vi "Mérésképernyő UI engedélyezés.vi"(8 "Error In":errorcluster, 10 "Felhasználói szint":string, 11 "UI Data":T1) -> (0 "Error Out":errorcluster, 3 "UI Data out":T1)   [LabVIEW 2014]
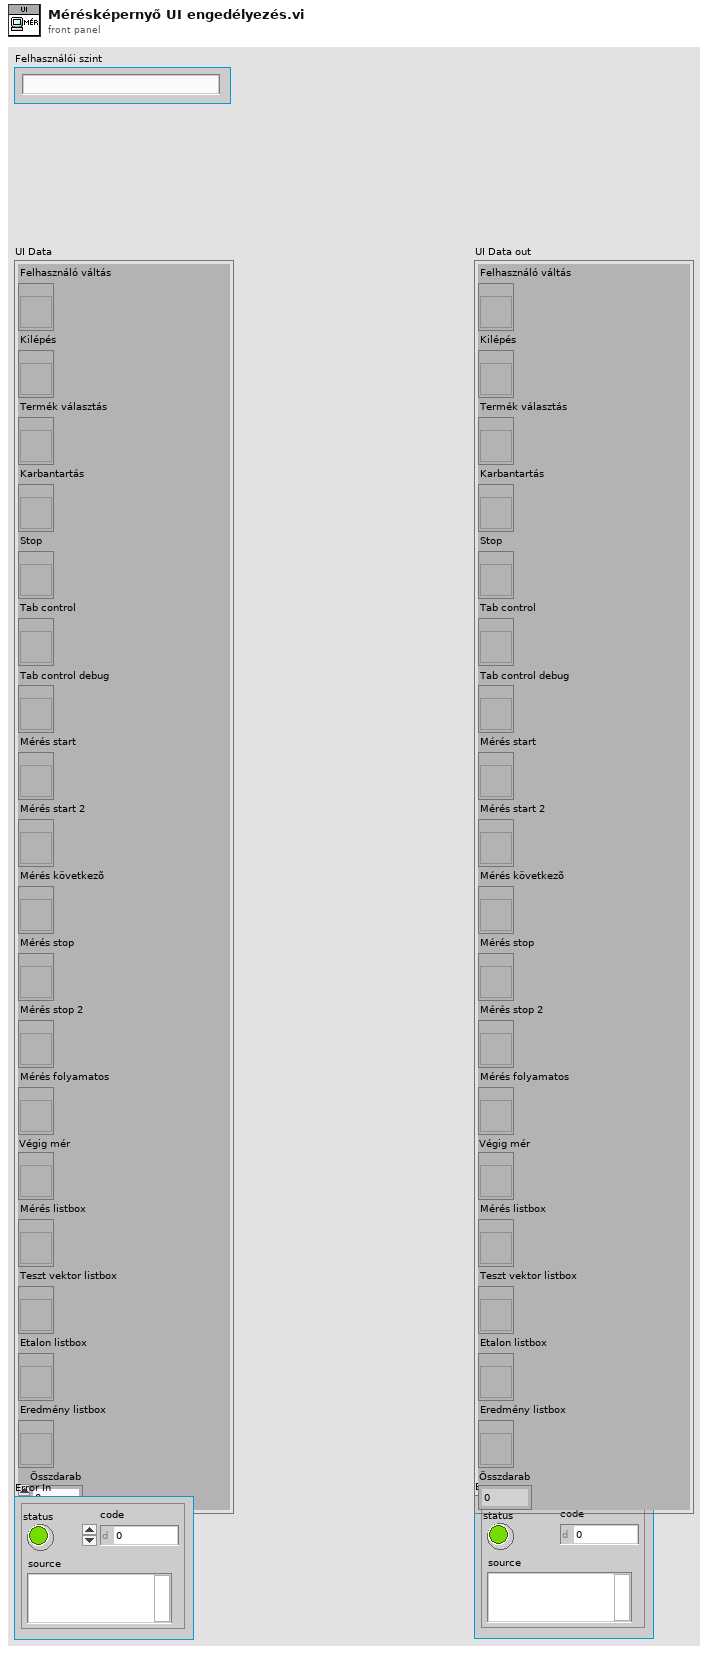
[diagram p1: front panel]
types:
  T1 = typedef "Fõképernyõ references.ctl" = cluster{"Felhasználó váltás":refnum<vi>, "Kilépés":refnum<vi>, "Termék választás":refnum<vi>, "Karbantartás":refnum<vi>, "Stop":refnum<vi>, "Tab control":refnum<vi>, "Tab control debug":refnum<vi>, "Mérés start":refnum<vi>, "Mérés start 2":refnum<vi>, "Mérés következõ":refnum<vi>, "Mérés stop":refnum<vi>, "Mérés stop 2":refnum<vi>, "Mérés folyamatos":refnum<vi>, "Végig mér":refnum<vi>, "Mérés listbox":refnum<vi>, "Teszt vektor listbox":refnum<vi>, "Etalon listbox":refnum<vi>, "Eredmény listbox":refnum<vi>, "Összdarab":i64}
  T2 = enum8{"Enabled", "Disabled", "Disabled and Grayed Out"}
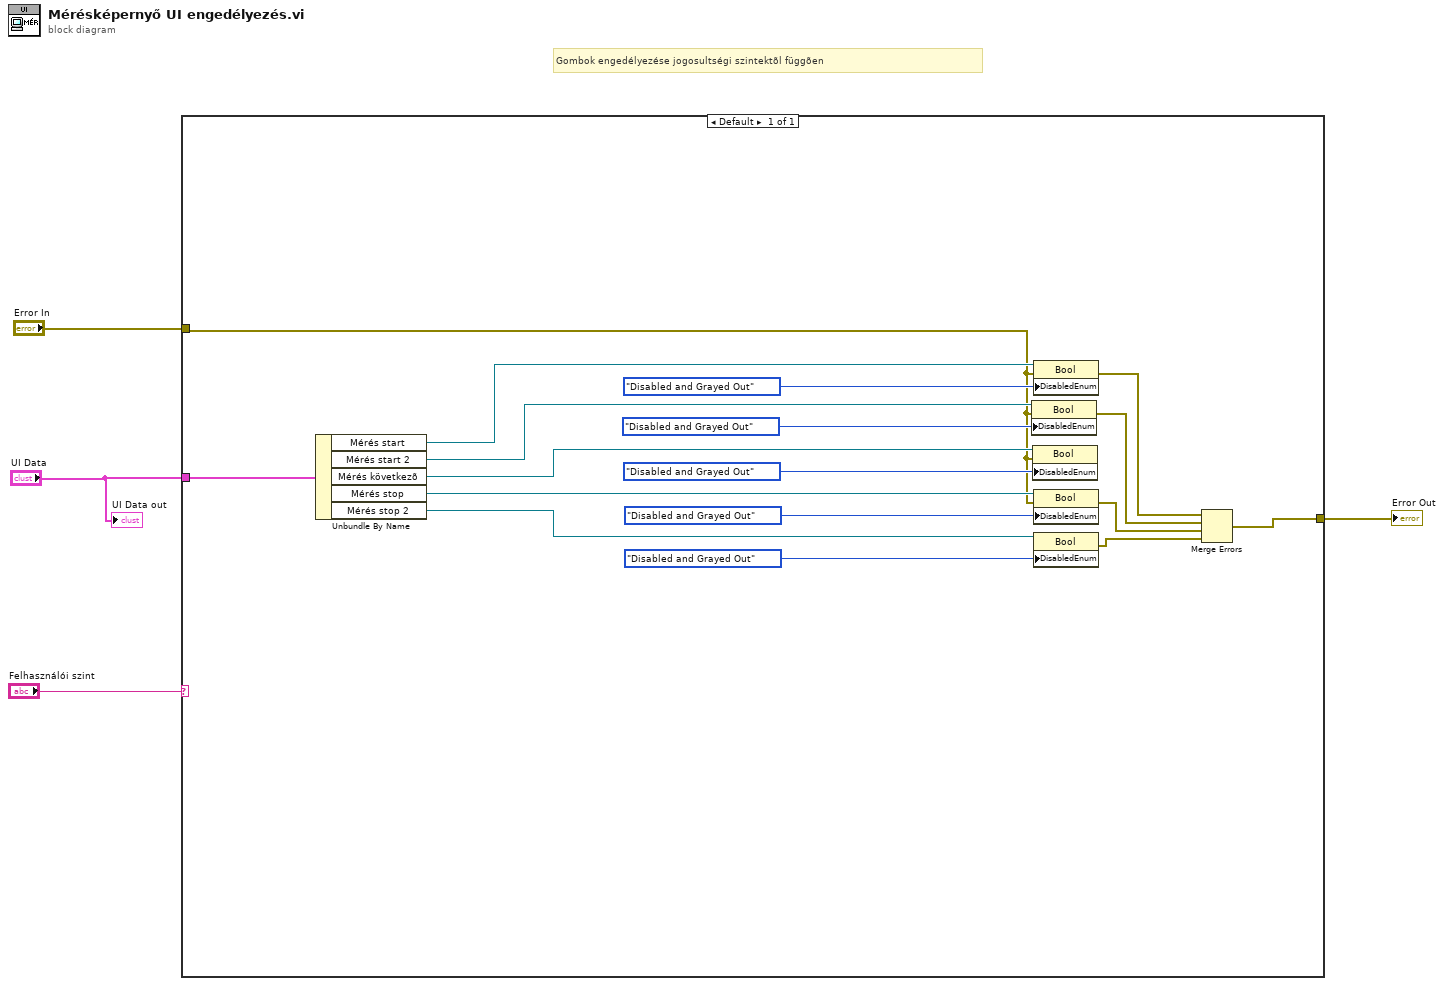
[diagram p0: block diagram]
diagram:
  # "Gombok engedélyezése jogosultségi szintektõl függõen"
  n1 = case shown="Default" "Felhasználói szint" {
    tunnel: [w10] -> w4
    tunnel: "UI Data" -> [w8]
    tunnel: "Error In" -> [w9]
    frame Default {
      n2 = Unbundle By Name(w8) -> ("Mérés start"=w19:refnum<vi>, "Mérés start 2"=w18:refnum<vi>, "Mérés következõ"=w17:refnum<vi>, "Mérés stop"=w15:refnum<vi>, "Mérés stop 2"=w6:refnum<vi>)
      n3 = property on="Property Node" class="Bool"(reference=w18, error in=w9, "DisabledEnum"=T2."Disabled and Grayed Out" ("Disabled")) -> (error out=w12:errorcluster)  [unwired: 1 out]
      n4 = property on="Property Node" class="Bool"(reference=w17, error in=w9, "DisabledEnum"=T2."Disabled and Grayed Out" ("Disabled")) -> ()  [unwired: 2 out]
      n5 = property on="Property Node" class="Bool"(reference=w19, error in=w9, "DisabledEnum"=T2."Disabled and Grayed Out" ("Disabled")) -> (error out=w13:errorcluster)  [unwired: 1 out]
      n6 = property on="Property Node" class="Bool"(reference=w15, error in=w9, "DisabledEnum"=T2."Disabled and Grayed Out" ("Disabled")) -> (error out=w11:errorcluster)  [unwired: 1 out]
      n7 = property on="Property Node" class="Bool"(reference=w6, "DisabledEnum"=T2."Disabled and Grayed Out" ("Disabled")) -> (error out=w5:errorcluster)  [unwired: 1 in, 1 out]
      n8 = Merge Errors(w13, w12, w11, w5) -> (w10:errorcluster)
    }
  }
  "Error Out" <- w4
  "UI Data out" <- "UI Data"
